vi "processString.vi"(8 "error in (no error)":errorcluster, 10 "Message in":string, 11 "Sent message in":refnum<class "BaseMessage.lvclass">) -> (0 "error out":errorcluster, 1 "found?":bool, 2 "response":T1, 3 "Sent message out":refnum<class "BaseMessage.lvclass">, 4 "isAck?":bool, 5 "Remaining buffer":string)   [LabVIEW 2025, in "BaseMessage.lvclass"]
doc: "Parses and interpretes the input string. If a complete packet from the remote host is found, \"found?\" should return TRUE. In that the case, the response should contain the type and the message data in the variant. \nIf the found message is an acknowledgement to the \"Sent message in\", the isAck? boolean should return TRUE.\nAnything left in the Message in string after the first message has been found should be returned in Remaining buffer"
uses:
  BaseMessage.lvclass
  response.ctl
  driver_status.ctl
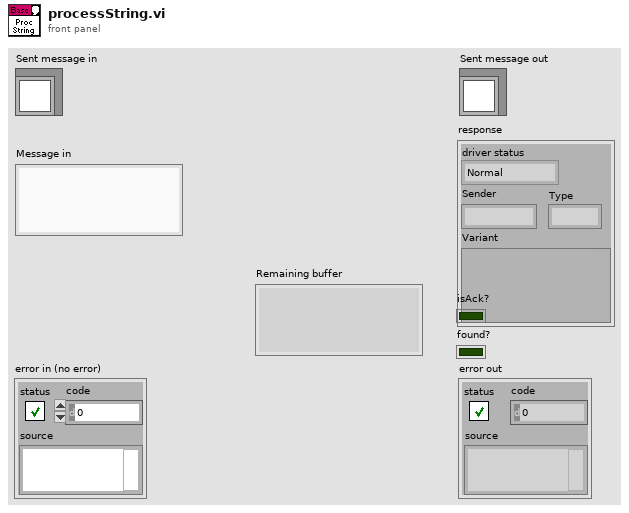
[diagram p1: front panel]
types:
  T1 = typedef "response.ctl" = cluster{"driver status":T2, "Sender":string, "Type":i32, "Variant":variant}
  T2 = typedef "driver_status.ctl" = enum16{"Normal", "Startup", "Connection lost", "Reconnected", "Timeout", "Idle", "Busy"}
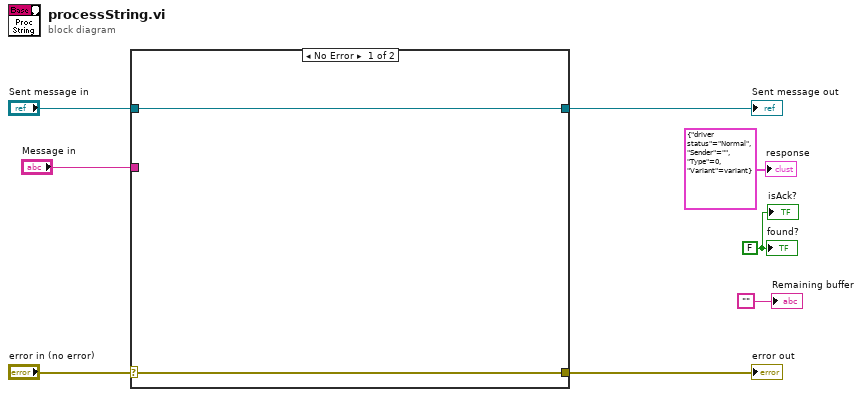
[diagram p0: block diagram]
diagram:
  w4 = FALSE ("found?")
  n1 = case shown="No Error" "error in (no error)" {
    selector: "error in (no error)" -> [w9 w12]
    tunnel: [w9 w12] -> w7
    tunnel: [w10 w11] -> w5
    tunnel: "Sent message in" -> [w10 w11]
    tunnel: "Message in" -> [_ _]
    frame No Error {
    }
    frame Error {
    }
  }
  "error out" <- w7
  "Sent message out" <- w5
  "response" <- T1 {"driver status"=enum."Normal", "Sender"="", "Type"=0, "Variant"=variant} ("response")
  "isAck?" <- w4
  "found?" <- w4
  "Remaining buffer" <- ""
